vi "UI.vi"() -> ()   [LabVIEW 2016, in "潮位站数据传输.lvlib"]
panel:
  in  "记录报文":bool
  out "数据大小":i32
  out "数据上传中":bool
  out "当前时间":timestamp
  out "error out":errorcluster
  out "数据查表起始时间":T1
  in  "数据补传":bool caption="确定"
  out "读取报文显示":string
  out "发送报文显示":string
  out "通信状态":bool
  in  "配置信息":T2
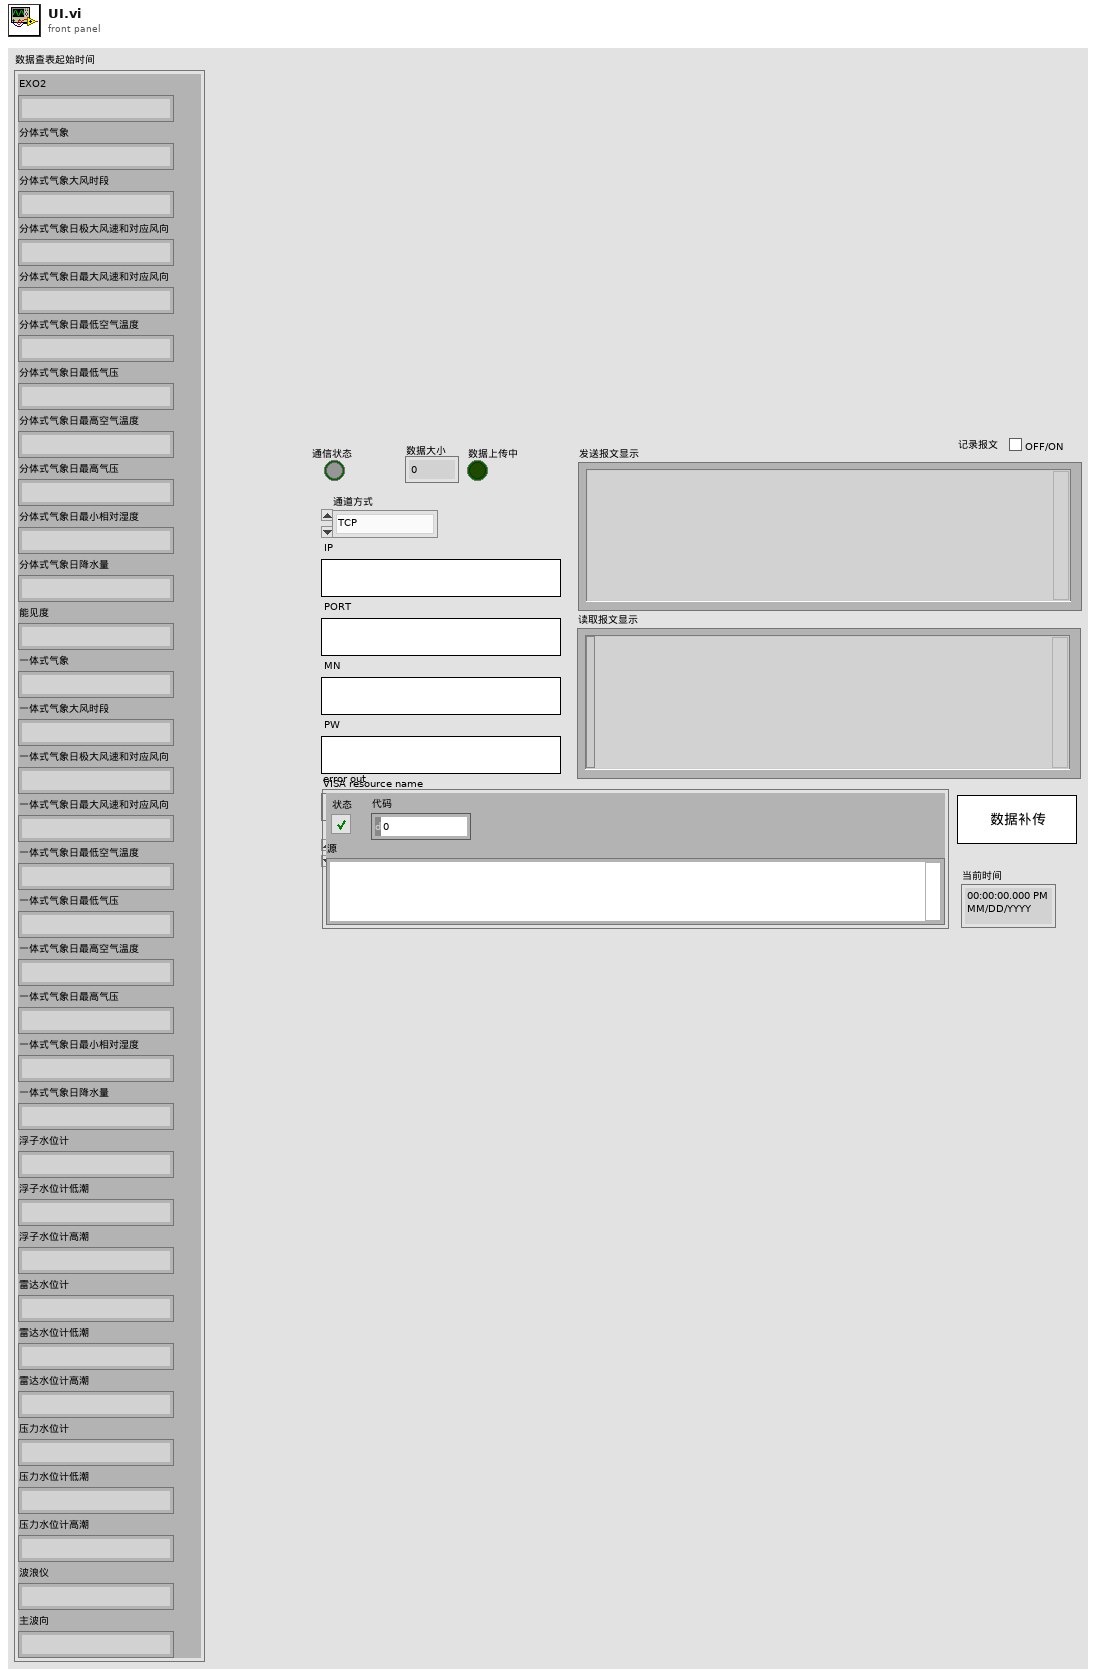
[diagram p1: front panel]
types:
  T1 = cluster{"EXO2":string, "分体式气象":string, "分体式气象大风时段":string, "分体式气象日极大风速和对应风向":string, "分体式气象日最大风速和对应风向":string, "分体式气象日最低空气温度":string, "分体式气象日最低气压":string, "分体式气象日最高空气温度":string, "分体式气象日最高气压":string, "分体式气象日最小相对湿度":string, "分体式气象日降水量":string, "能见度":string, "一体式气象":string, "一体式气象大风时段":string, "一体式气象日极大风速和对应风向":string, "一体式气象日最大风速和对应风向":string, "一体式气象日最低空气温度":string, "一体式气象日最低气压":string, "一体式气象日最高空气温度":string, "一体式气象日最高气压":string, "一体式气象日最小相对湿度":string, "一体式气象日降水量":string, "浮子水位计":string, "浮子水位计低潮":string, "浮子水位计高潮":string, "雷达水位计":string, "雷达水位计低潮":string, "雷达水位计高潮":string, "压力水位计":string, "压力水位计低潮":string, "压力水位计高潮":string, "波浪仪":string, "主波向":string}
  T2 = cluster{"通道方式":enum16{"TCP", "serial"}, "IP":string, "PORT":string, "MN":string, "PW":string, "VISA resource name":refnum<visa-resource-name>, "baud rate":u32}
  T3 = typedef "LVDateTimeRec.ctl" = cluster{"秒数的小数部分":dbl, "秒":i32, "分":i32, "时":i32, "日":i32, "月":i32, "年":i32, "天数（周）":i32, "天数（年）":i32, "DST":i32}
  T4 = cluster{"[0]":string, "[1]":string, "[2]":string, "[3]":string, "[4]":string, "[5]":string, "[6]":string, "[7]":string, "[8]":string, "[9]":string, "[10]":string, "[11]":string, "[12]":string, "[13]":string, "[14]":string, "[15]":string, "[16]":string, "[17]":string, "[18]":string, "[19]":string, "[20]":string, "[21]":string, "[22]":string, "[23]":string, "[24]":string, "[25]":string, "[26]":string, "[27]":string, "[28]":string, "[29]":string, "[30]":string, "[31]":string, "[32]":string}
  T5 = cluster{"枚举":enum16{"打开连接", "发送数据", "读取数据", "数据处理", "关闭连接"}, "data":string}
  T6 = cluster{"枚举":enum16{"TCP", "serial"}, "IP":string, "PORT":string, "MN":string, "PW":string, "VISA resource name":refnum<visa-resource-name>, "baud rate":u32}
  T7 = typedef "潮位站数据传输.lvlib/data_in.ctl" = cluster{"PW":string, "MN":string, "table输入":T8, "数据发送次数":i32, "枚举":enum16{"返回请求应答", "上传数据", "返回执行结果"}, "type":T9, "因子编码&数据类型":cluster{"因子编码":string, "数据类型":T10}[]}
  T8 = typedef "潮位站数据传输.lvlib/table.ctl" = string
  T9 = typedef "潮位站数据传输.lvlib/Type.ctl" = string
  T10 = typedef "潮位站数据传输.lvlib/data_type.ctl" = string
  T11 = cluster{"table":string, "columns":string[], "condition":string, "data_in":T7}
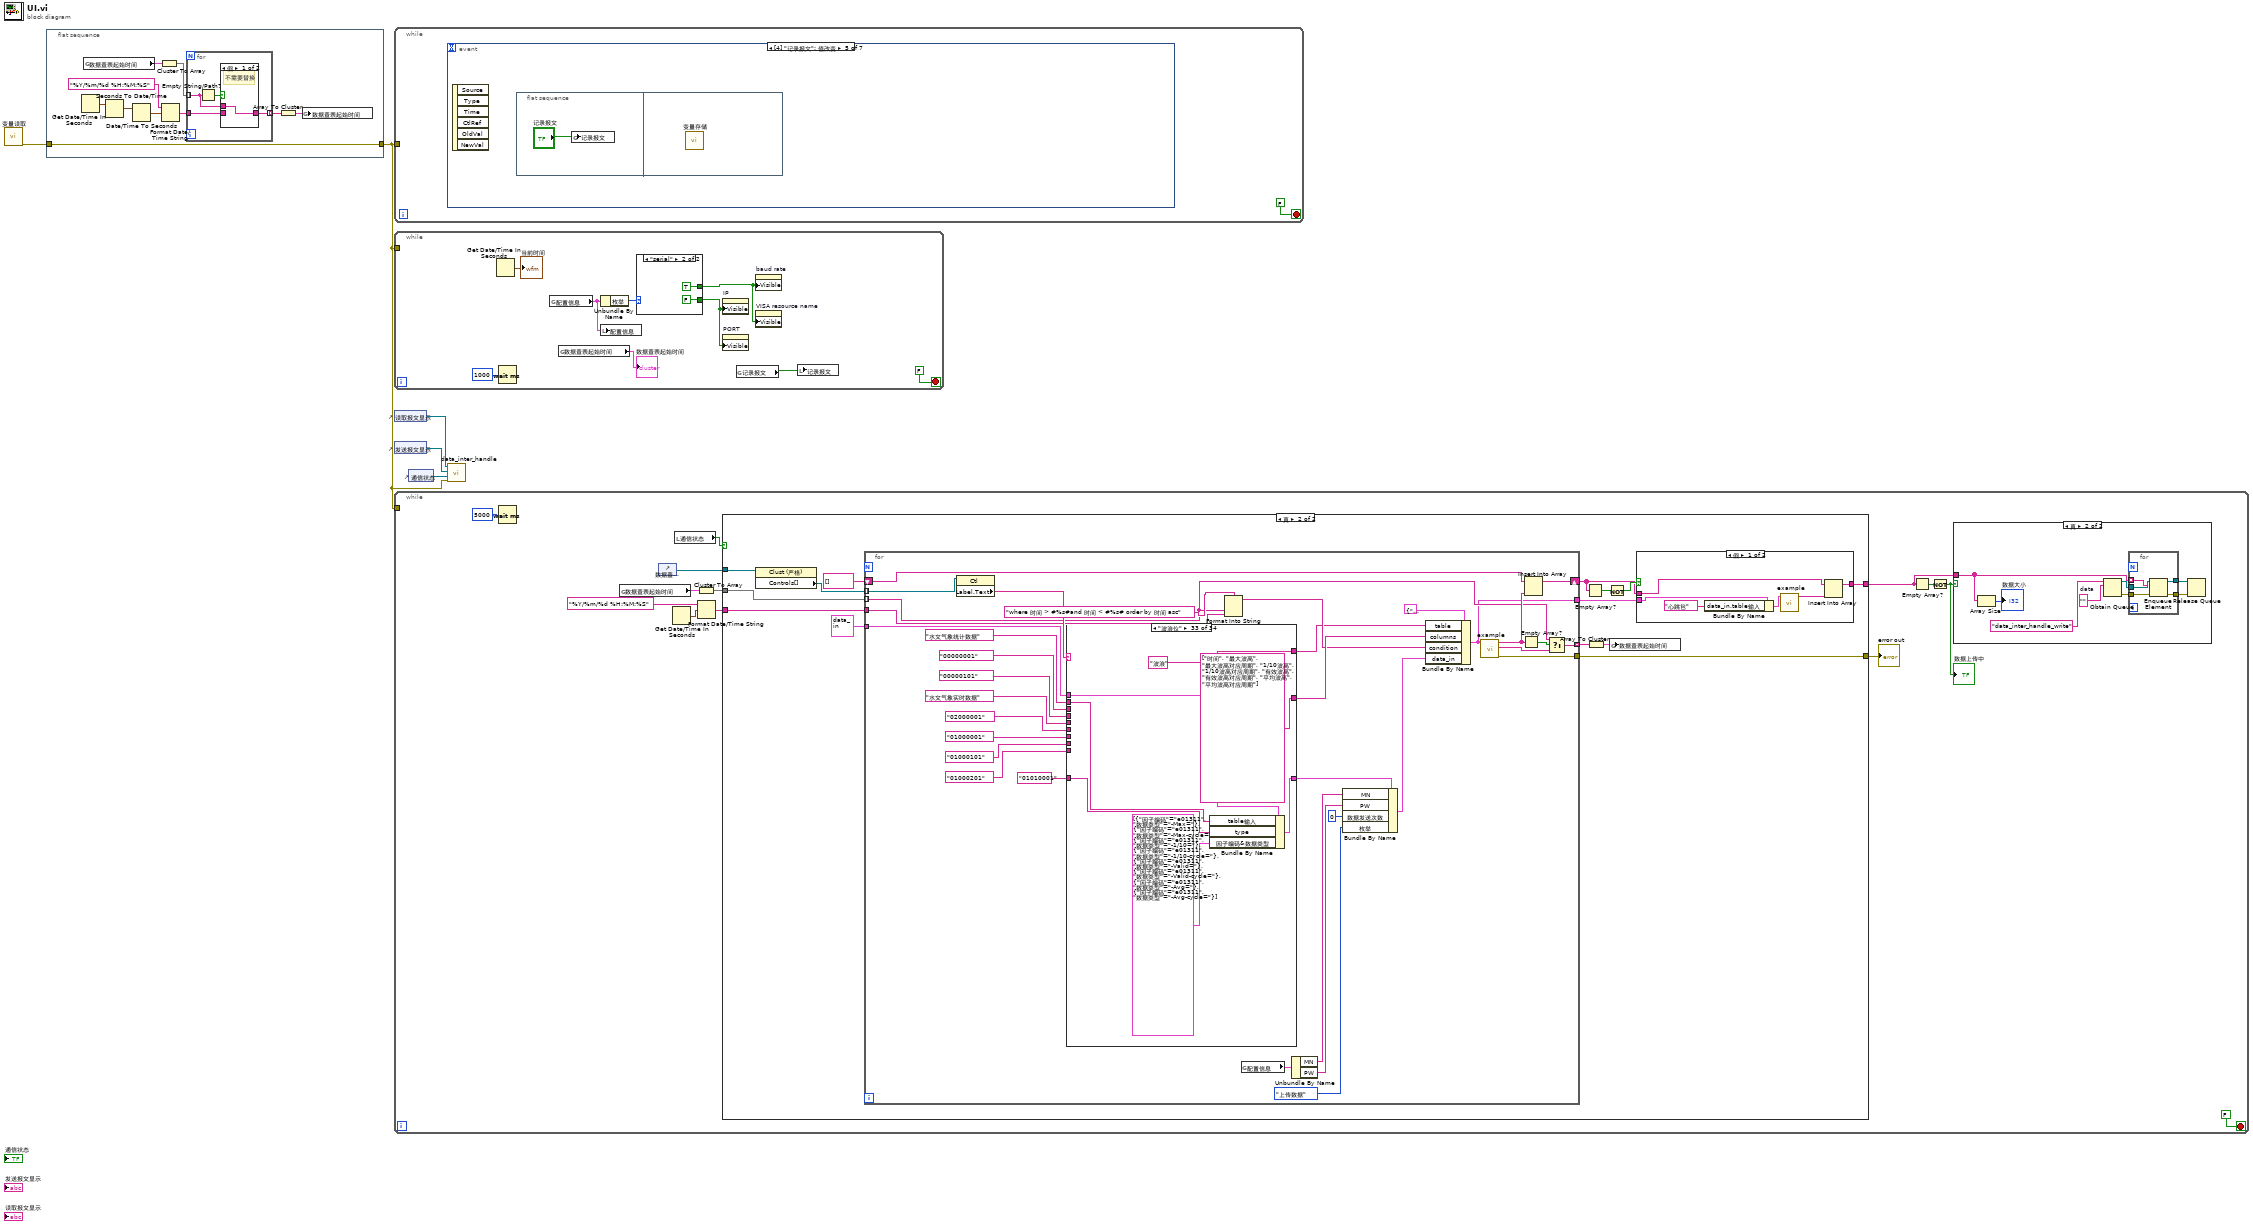
[diagram p0: block diagram]
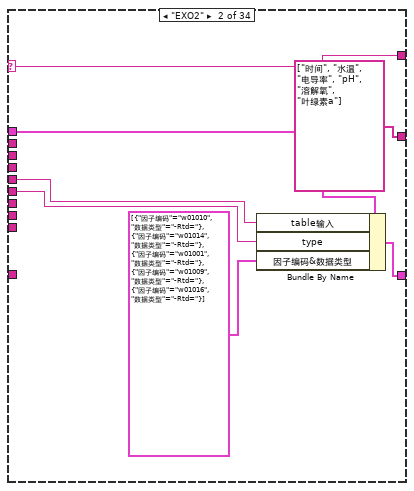
[diagram p6: hidden frame]
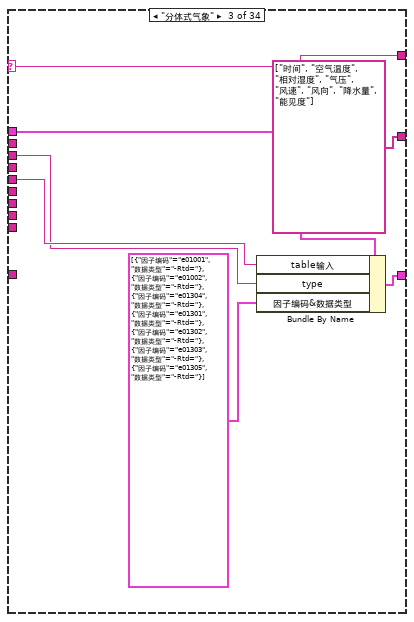
[diagram p7: hidden frame]
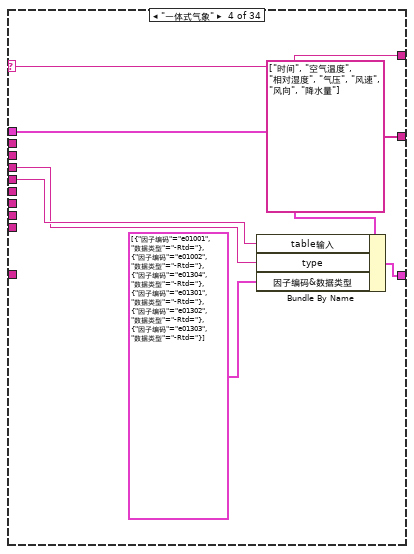
[diagram p8: hidden frame]
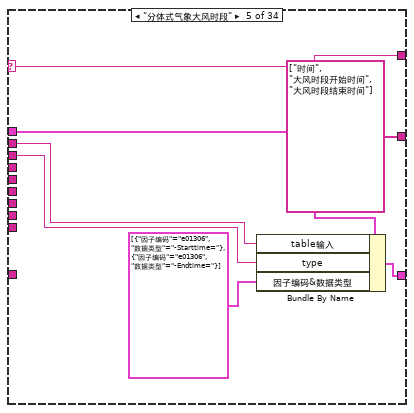
[diagram p9: hidden frame]
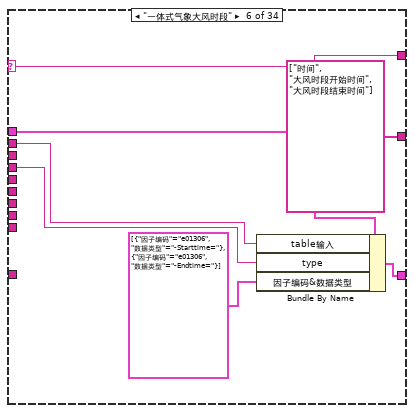
[diagram p10: hidden frame]
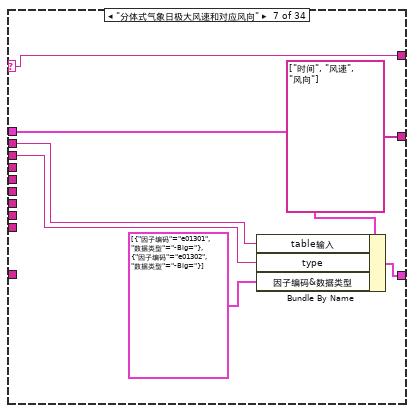
[diagram p11: hidden frame]
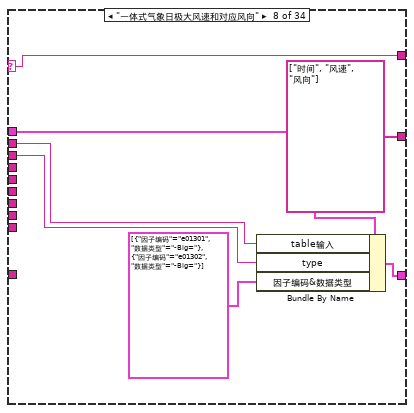
[diagram p12: hidden frame]
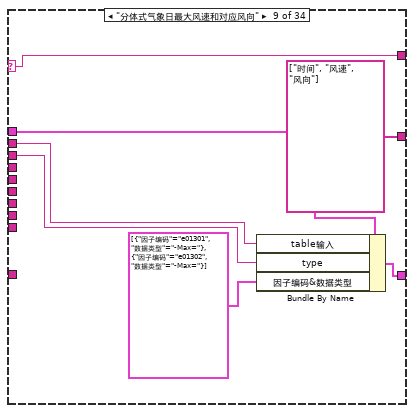
[diagram p13: hidden frame]
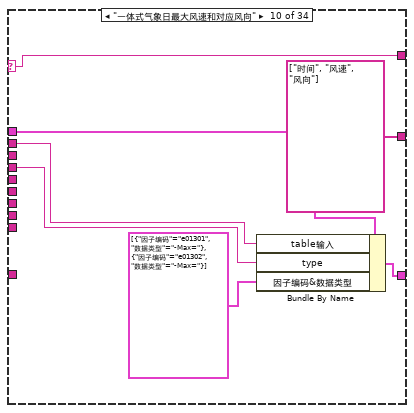
[diagram p14: hidden frame]
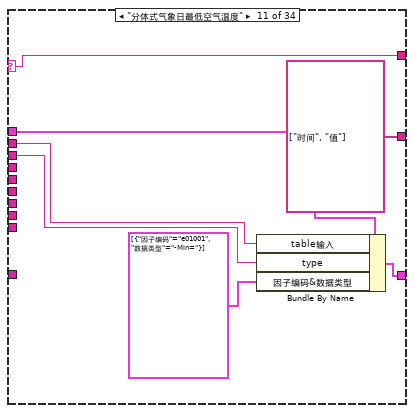
[diagram p15: hidden frame]
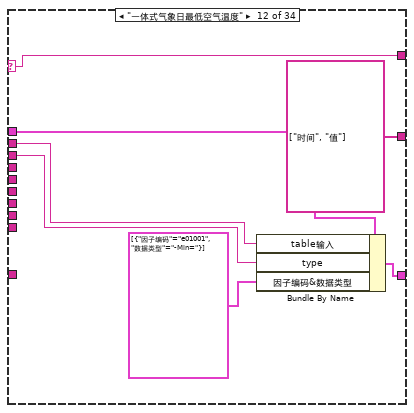
[diagram p16: hidden frame]
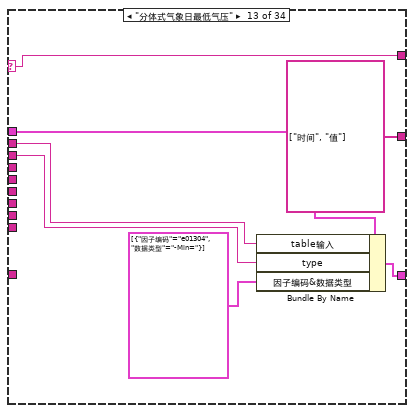
[diagram p17: hidden frame]
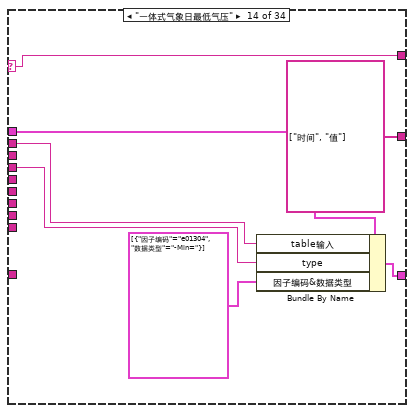
[diagram p18: hidden frame]
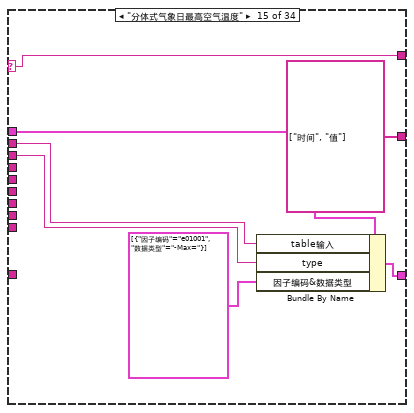
[diagram p19: hidden frame]
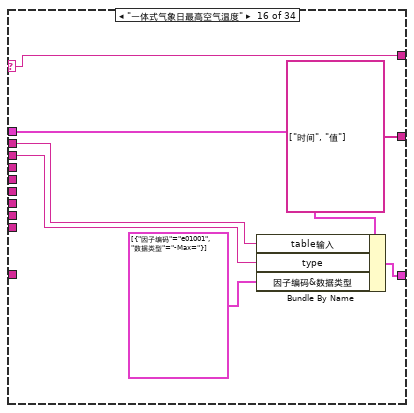
[diagram p20: hidden frame]
diagram:
  n1 = call "变量读取.vi"() -> ("错误输出"=w5:errorcluster)  [unwired: 11 in]
  n2 = flat-sequence {
    tunnel: w5 -> [w8]
    tunnel: [w8] -> w4
    frame #0 {
      n3 = Get Date/Time In Seconds() -> (seconds since 1Jan1904=w7:timestamp)
      n4 = global read "断电保存全局.vi" "数据查表起始时间"() -> (w13:T1)
      n5 = Seconds To Date/Time(time stamp (now)=w7) -> (date time rec=w6:T3)  [unwired: 1 in]
      n6 = Date/Time To Seconds(2:w6) -> (0:w11:timestamp)  [unwired: 1 in]
      n7 = Cluster To Array(cluster=w13) -> (array=w14:string[])
      n8 = Format Date/Time String(time format string (%c)="%Y/%m/%d %H:%M:%S" ("时间格式字符串(%c)"), seconds (now)=w11) -> (date/time string=w10:string)  [unwired: 1 in]
      n9 = for {
        tunnel: w14 -> [w16] mode=indexing
        tunnel: w10 -> [w18]
        tunnel: [w17] -> w15 mode=indexing
        n10 = Empty String/Path?(string/path=w16) -> (empty?=w19:bool)
        n11 = case shown="假" w19 {
          tunnel: w18 -> [_ w21]
          tunnel: [w20 w21] -> w17
          tunnel: w16 -> [w20 _]
          frame False {
            # "不需要替换"
          }
          frame True {
            # "空字符串，替换"
          }
        }
      }
      n12 = Array To Cluster(array=w15) -> (cluster=w9:T4)
      n13 = global write "断电保存全局.vi" "数据查表起始时间"(w9) -> ()
    }
  }
  n14 = while {
    tunnel: w4 -> [_]
    stop <- FALSE stop-if-true
    n15 = event shown="[4] \"记录报文\": 值改变" {
      selector: _ -> [_ _ _ _ _ _ _]
      dyn-events: _ -> [_ _ _ _ _ _ _]
      timeout: _ -> [_ _ _ _ _ _ _]
      event Timeout {
        n16 = event-data() -> ()  [unwired: 1 in, 3 out]
      }
      event "配置信息.IP", "配置信息.PORT": Mouse Down {
        n17 = event-data() -> ("CtlRef"=w31:refnum<vi>)  [unwired: 1 in, 7 out]
        n18 = property class="Str"(reference=w31) -> (reference out=w24:refnum<vi>, "Value"=w30:string)  [unwired: 1 in, 1 out]
        n19 = call "IP键盘.vi"("OldNumber"=w30) -> ("NewNumber"=w23:string)
        n20 = String Length(string=w23) -> (length=w29:i32)
        n21 = Less Or Equal?(x=w29, y=50) -> (x <= y?=w27:bool)
        n22 = case shown="假" w27 {
          tunnel: w24 -> [w32 w36]
          tunnel: w23 -> [_ w35]
          tunnel: [w32 w36] -> w26
          tunnel: ["127.0.0.1" w35] -> w25
          frame False {
            n23 = One Button Dialog(message="超过ipv4最大长度限制,请重新输入!" ("消息")) -> ()  [unwired: 1 in, 1 out]
          }
          frame True {
          }
        }
        n24 = property class="Str"(reference=w26, "Val(Sgnl)"=w25) -> ()  [unwired: 1 in, 2 out]
      }
      event "配置信息.baud rate": Mouse Down {
        n25 = event-data() -> ("CtlRef"=w40:refnum<vi>)  [unwired: 1 in, 7 out]
        n26 = property class="DigNum (严格)"(reference=w40) -> (reference out=w38:refnum<vi>, "Value"=w39:u32)  [unwired: 1 in, 1 out]
        n27 = call "数字键盘.vi"("OldNumber"=w39) -> ("NewNumber"=w37:sgl)
        n28 = property class="DigNum (严格)"(reference=w38, "Val(Sgnl)"=w37) -> ()  [unwired: 1 in, 2 out]
      }
      event "配置信息": Value Change {
        n29 = event-data() -> ()  [unwired: 1 in, 6 out]
        n30 = flat-sequence {
          frame #0 {
            n31 = global write "断电保存全局.vi" "配置信息"("配置信息") -> ()
          }
          frame #1 {
            w46 = T5 {"枚举"=enum."打开连接", "data"=""}
            n32 = call "变量存储.vi"() -> ()  [unwired: 12 in]
            n33 = Bundle By Name(cluster=w46, "枚举"=enum16{"打开连接", "发送数据", "读取数据", "数据处理", "关闭连接"}."关闭连接") -> (w45:T5)
            n34 = Obtain Queue(name (unnamed)="data_inter_handle" ("名称（未命名）"), element data type=w46) -> (queue out=w48:refnum<queue>, error out=w47:errorcluster)  [unwired: 3 in, 1 out]
            n35 = Enqueue Element(queue=w48, element=w45, error in (no error)=w47) -> (queue out=w42:refnum<queue>, error out=w43:errorcluster)  [unwired: 1 in, 1 out]
            n36 = Release Queue(queue=w42, error in (no error)=w43) -> ()  [unwired: 1 in, 3 out]
          }
        }
      }
      event "记录报文": Value Change {
        n37 = event-data() -> ()  [unwired: 1 in, 6 out]
        n38 = flat-sequence {
          frame #0 {
            n39 = global write "断电保存全局.vi" "记录报文"("记录报文") -> ()
          }
          frame #1 {
            n40 = call "变量存储.vi"() -> ()  [unwired: 12 in]
          }
        }
      }
      event "数据补传": Value Change {
        n41 = event-data() -> ()  [unwired: 1 in, 6 out]
        n42 = call "数据补传对话框.vi"() -> ("输出"=w52:bool, "时间OUT"=w51:timestamp)  [unwired: 10 in]
        n43 = case shown="真" w52 {
          tunnel: w51 -> [_ w57]
          frame False {
          }
          frame True {
            n44 = Format Date/Time String(time format string (%c)="%Y/%m/%d %H:%M:%S" ("时间格式字符串(%c)"), seconds (now)=w57) -> (date/time string=w54:string)  [unwired: 1 in]
            n45 = Initialize Array(w54, 33 ("维数大小")) -> (w53:string[])
            n46 = Array To Cluster(array=w53) -> (cluster=w55:T4)
            n47 = global write "断电保存全局.vi" "数据查表起始时间"(w55) -> ()
          }
        }
      }
      event Panel Close {
        n48 = event-data() -> ()  [unwired: 1 in, 4 out]
        n49 = Quit LabVIEW(quit? (T)=TRUE ("退出？(T)")) -> ()
      }
    }
  }
  n50 = while {
    tunnel: w4 -> [_]
    stop <- FALSE stop-if-true
    n51 = Get Date/Time In Seconds() -> (seconds since 1Jan1904=→"当前时间":timestamp)
    n52 = Wait (ms)(milliseconds to wait=u32 1000 ("等待时间（毫秒）")) -> ()  [unwired: 1 out]
    n53 = global read "断电保存全局.vi" "配置信息"() -> (w64:T6)
    n54 = global read "断电保存全局.vi" "数据查表起始时间"() -> (→"数据查表起始时间":T1)
    n55 = local write "配置信息"(w64) -> ()
    n56 = Unbundle By Name(w64) -> ("枚举"=w63:enum16{"TCP", "serial"})
    n57 = case shown="\"serial\"" w63 {
      tunnel: [TRUE FALSE] -> w62
      tunnel: [FALSE TRUE] -> w61
      frame "TCP", Default {
      }
      frame "serial" {
      }
    }
    n58 = property on="IP" class="Str"("Visible"=w62) -> ()  [unwired: 2 in, 2 out]
    n59 = property on="PORT" class="Str"("Visible"=w62) -> ()  [unwired: 2 in, 2 out]
    n60 = global read "断电保存全局.vi" "记录报文"() -> (w60:bool)
    n61 = property on="baud rate" class="DigNum (严格)"("Visible"=w61) -> ()  [unwired: 2 in, 2 out]
    n62 = property on="VISA resource name" class="VISAName"("Visible"=w61) -> ()  [unwired: 2 in, 2 out]
    n63 = local write "记录报文"(w60) -> ()
  }
  n64 = control-ref of="读取报文显示"() -> (w2:refnum<vi>)
  n65 = control-ref of="发送报文显示"() -> (w3:refnum<vi>)
  n66 = while {
    tunnel: w4 -> [_]
    stop <- FALSE stop-if-true
    n67 = Wait (ms)(milliseconds to wait=u32 5000 ("等待时间（毫秒）")) -> ()  [unwired: 1 out]
    n68 = global read "断电保存全局.vi" "数据查表起始时间"() -> (w83:T1)
    n69 = control-ref of="数据查表起始时间"() -> (w77:refnum<vi>)
    n70 = Get Date/Time In Seconds() -> (seconds since 1Jan1904=w79:timestamp)
    n71 = local read "通信状态"() -> (w74:bool)
    n72 = Cluster To Array(cluster=w83) -> (array=w82:string[])
    n73 = Format Date/Time String(time format string (%c)="%Y/%m/%d %H:%M:%S" ("时间格式字符串(%c)"), seconds (now)=w79) -> (date/time string=w80:string)  [unwired: 1 in]
    n74 = case shown="真" w74 {
      tunnel: w82 -> [_ w99]
      tunnel: w80 -> [_ w98]
      tunnel: [_ w87] -> w73
      tunnel: w77 -> [_ w97]
      tunnel: [_ w95] -> w76
      frame False {
      }
      frame True {
        n75 = property class="Clust (严格)"(reference=w97) -> ("Controls[]"=w96:refnum<vi>[])  [unwired: 1 in, 2 out]
        n76 = for {
          tunnel: w99 -> [w124] mode=indexing
          tunnel: w96 -> [w140] mode=indexing
          tunnel: w98 -> [w130]
          shift-right: [w127] -> w88
          shift-left: string[] [] ("message") -> [w128]
          tunnel: [w122] -> w92 mode=indexing
          tunnel: [w121] -> w95
          tunnel: T7 {"PW"="123456", "MN"="TEST001", "table输入"="心跳包", "数据发送次数"=0, "枚举"=enum."上传数据", "type"="00000001", "因子编码&数据类型"=[{"因子编码"="e01306", "数据类型"="-Starttime="}, {"因子编码"="e01307", "数据类型"="-Endtime="}]} ("data_in") -> [w119]
          tunnel: [w110] -> w86
          n77 = property class="Ctl"(reference=w140) -> ("Label.Text"=w139:string)  [unwired: 1 in, 2 out]
          n78 = case shown="\"波浪仪\"" w139 {
            selector: w139 -> [w141 w142 w149 w156 w163 w170 w177 w184 w191 w198 w205 w212 w219 w226 w233 w240 w247 w254 w261 w268 w275 w282 w289 w296 w303 w310 w317 w324 w331 w338 w345 w352 _ _]
            tunnel: [_ string[] ["时间", "水温", "电导率", "pH", "溶解氧", "叶绿素a"] ("columns") string[] ["时间", "空气温度", "相对湿度", "气压", "风速", "风向", "降水量", "能见度"] ("columns") string[] ["时间", "空气温度", "相对湿度", "气压", "风速", "风向", "降水量"] ("columns") string[] ["时间", "大风时段开始时间", "大风时段结束时间"] ("columns") string[] ["时间", "大风时段开始时间", "大风时段结束时间"] ("columns") string[] ["时间", "风速", "风向"] ("columns") string[] ["时间", "风速", "风向"] ("columns") string[] ["时间", "风速", "风向"] ("columns") string[] ["时间", "风速", "风向"] ("columns") string[] ["时间", "值"] ("columns") string[] ["时间", "值"] ("columns") string[] ["时间", "值"] ("columns") string[] ["时间", "值"] ("columns") string[] ["时间", "值"] ("columns") string[] ["时间", "值"] ("columns") string[] ["时间", "值"] ("columns") string[] ["时间", "值"] ("columns") string[] ["时间", "值"] ("columns") string[] ["时间", "值"] ("columns") string[] ["时间", "值"] ("columns") string[] ["时间", "值"] ("columns") string[] ["时间", "60秒能见度"] ("columns") string[] ["时间", "潮高"] ("columns") string[] ["时间", "潮高"] ("columns") string[] ["时间", "潮高"] ("columns") string[] ["时间", "潮高"] ("columns") string[] ["时间", "潮高"] ("columns") string[] ["时间", "潮高"] ("columns") string[] ["时间", "潮高"] ("columns") string[] ["时间", "潮高"] ("columns") string[] ["时间", "潮高"] ("columns") string[] ["时间", "最大波高", "最大波高对应周期", "1/10波高", "1/10波高对应周期", "有效波高", "有效波高对应周期", "平均波高", "平均波高对应周期"] ("columns") string[] ["时间", "主波向"] ("columns")] -> w138
            tunnel: w119 -> [_ w147 w154 w161 w168 w175 w182 w189 w196 w203 w210 w217 w224 w231 w238 w245 w252 w259 w266 w273 w280 w287 w294 w301 w308 w315 w322 w329 w336 w343 w350 w357 w364 w372]
            tunnel: [_ w146 w153 w160 w167 w174 w181 w188 w195 w202 w209 w216 w223 w230 w237 w244 w251 w258 w265 w272 w279 w286 w293 w300 w307 w314 w321 w328 w335 w342 w349 w356 w363 w371] -> w108
            tunnel: T9 "00000001" ("type") -> [_ _ w150 _ w165 _ w179 w185 w193 _ w207 w214 w221 _ w235 w242 w249 _ w263 _ w276 _ w290 _ _ _ _ _ _ _ _ _ _ _]
            tunnel: T9 "00000101" ("type") -> [_ _ _ w157 _ w171 _ _ _ w200 _ _ _ w228 _ _ _ w256 _ w270 _ w284 _ _ _ _ _ _ _ _ _ _ _ _]
            tunnel: T9 "01000001" ("type") -> [_ _ _ _ _ _ _ _ _ _ _ _ _ _ _ _ _ _ _ _ _ _ _ w298 _ _ w318 _ _ w340 _ _ _ _]
            tunnel: T9 "01000101" ("type") -> [_ _ _ _ _ _ _ _ _ _ _ _ _ _ _ _ _ _ _ _ _ _ _ _ w305 _ _ w326 _ _ w346 _ _ _]
            tunnel: T9 "01000201" ("type") -> [_ _ _ _ _ _ _ _ _ _ _ _ _ _ _ _ _ _ _ _ _ _ _ _ _ w312 _ _ w332 _ _ w354 _ _]
            tunnel: T9 "02000001" ("type") -> [_ w143 _ _ _ _ _ _ _ _ _ _ _ _ _ _ _ _ _ _ _ _ _ _ _ _ _ _ _ _ _ _ _ _]
            tunnel: T8 "水文气象实时数据" ("table输入") -> [_ w144 w151 w158 _ _ _ _ _ _ _ _ _ _ _ _ _ _ _ _ _ _ w291 w297 w304 w311 _ _ _ _ _ _ _ w367]
            tunnel: T8 "水文气象统计数据" ("table输入") -> [_ _ _ _ w164 w172 w178 w186 w192 w199 w206 w213 w220 w227 w234 w241 w248 w255 w262 w269 w277 w283 _ _ _ _ w319 w325 w333 w339 w347 w353 w361 _]
            tunnel: T9 "01010001" ("type") -> [_ _ _ _ _ _ _ _ _ _ _ _ _ _ _ _ _ _ _ _ _ _ _ _ _ _ _ _ _ _ _ _ w360 w369]
            tunnel: [w141 w142 w149 w156 w163 w170 w177 w184 w191 w198 w205 w212 w219 w226 w233 w240 w247 w254 w261 w268 w275 w282 w289 w296 w303 w310 w317 w324 w331 w338 w345 w352 "波浪" "波浪"] -> w107
            frame "假", Default {
            }
            frame "EXO2" {
              n79 = Bundle By Name(cluster=w147, "table输入"=w144, "type"=w143, "因子编码&数据类型"=cluster{"因子编码":string, "数据类型":string}[] [{"因子编码"="w01010", "数据类型"="-Rtd="}, {"因子编码"="w01014", "数据类型"="-Rtd="}, {"因子编码"="w01001", "数据类型"="-Rtd="}, {"因子编码"="w01009", "数据类型"="-Rtd="}, {"因子编码"="w01016", "数据类型"="-Rtd="}]) -> (w146:T7)
            }
            frame "分体式气象" {
              n80 = Bundle By Name(cluster=w154, "table输入"=w151, "type"=w150, "因子编码&数据类型"=cluster{"因子编码":string, "数据类型":string}[] [{"因子编码"="e01001", "数据类型"="-Rtd="}, {"因子编码"="e01002", "数据类型"="-Rtd="}, {"因子编码"="e01304", "数据类型"="-Rtd="}, {"因子编码"="e01301", "数据类型"="-Rtd="}, {"因子编码"="e01302", "数据类型"="-Rtd="}, {"因子编码"="e01303", "数据类型"="-Rtd="}, {"因子编码"="e01305", "数据类型"="-Rtd="}]) -> (w153:T7)
            }
            frame "一体式气象" {
              n81 = Bundle By Name(cluster=w161, "table输入"=w158, "type"=w157, "因子编码&数据类型"=cluster{"因子编码":string, "数据类型":string}[] [{"因子编码"="e01001", "数据类型"="-Rtd="}, {"因子编码"="e01002", "数据类型"="-Rtd="}, {"因子编码"="e01304", "数据类型"="-Rtd="}, {"因子编码"="e01301", "数据类型"="-Rtd="}, {"因子编码"="e01302", "数据类型"="-Rtd="}, {"因子编码"="e01303", "数据类型"="-Rtd="}]) -> (w160:T7)
            }
            frame "分体式气象大风时段" {
              n82 = Bundle By Name(cluster=w168, "table输入"=w164, "type"=w165, "因子编码&数据类型"=cluster{"因子编码":string, "数据类型":string}[] [{"因子编码"="e01306", "数据类型"="-Starttime="}, {"因子编码"="e01306", "数据类型"="-Endtime="}]) -> (w167:T7)
            }
            frame "一体式气象大风时段" {
              n83 = Bundle By Name(cluster=w175, "table输入"=w172, "type"=w171, "因子编码&数据类型"=cluster{"因子编码":string, "数据类型":string}[] [{"因子编码"="e01306", "数据类型"="-Starttime="}, {"因子编码"="e01306", "数据类型"="-Endtime="}]) -> (w174:T7)
            }
            frame "分体式气象日极大风速和对应风向" {
              n84 = Bundle By Name(cluster=w182, "table输入"=w178, "type"=w179, "因子编码&数据类型"=cluster{"因子编码":string, "数据类型":string}[] [{"因子编码"="e01301", "数据类型"="-Big="}, {"因子编码"="e01302", "数据类型"="-Big="}]) -> (w181:T7)
            }
            frame "一体式气象日极大风速和对应风向" {
              n85 = Bundle By Name(cluster=w189, "table输入"=w186, "type"=w185, "因子编码&数据类型"=cluster{"因子编码":string, "数据类型":string}[] [{"因子编码"="e01301", "数据类型"="-Big="}, {"因子编码"="e01302", "数据类型"="-Big="}]) -> (w188:T7)
            }
            frame "分体式气象日最大风速和对应风向" {
              n86 = Bundle By Name(cluster=w196, "table输入"=w192, "type"=w193, "因子编码&数据类型"=cluster{"因子编码":string, "数据类型":string}[] [{"因子编码"="e01301", "数据类型"="-Max="}, {"因子编码"="e01302", "数据类型"="-Max="}]) -> (w195:T7)
            }
            frame "一体式气象日最大风速和对应风向" {
              n87 = Bundle By Name(cluster=w203, "table输入"=w199, "type"=w200, "因子编码&数据类型"=cluster{"因子编码":string, "数据类型":string}[] [{"因子编码"="e01301", "数据类型"="-Max="}, {"因子编码"="e01302", "数据类型"="-Max="}]) -> (w202:T7)
            }
            frame "分体式气象日最低空气温度" {
              n88 = Bundle By Name(cluster=w210, "table输入"=w206, "type"=w207, "因子编码&数据类型"=cluster{"因子编码":string, "数据类型":string}[] [{"因子编码"="e01001", "数据类型"="-Min="}]) -> (w209:T7)
            }
            frame "一体式气象日最低空气温度" {
              n89 = Bundle By Name(cluster=w217, "table输入"=w213, "type"=w214, "因子编码&数据类型"=cluster{"因子编码":string, "数据类型":string}[] [{"因子编码"="e01001", "数据类型"="-Min="}]) -> (w216:T7)
            }
            frame "分体式气象日最低气压" {
              n90 = Bundle By Name(cluster=w224, "table输入"=w220, "type"=w221, "因子编码&数据类型"=cluster{"因子编码":string, "数据类型":string}[] [{"因子编码"="e01304", "数据类型"="-Min="}]) -> (w223:T7)
            }
            frame "一体式气象日最低气压" {
              n91 = Bundle By Name(cluster=w231, "table输入"=w227, "type"=w228, "因子编码&数据类型"=cluster{"因子编码":string, "数据类型":string}[] [{"因子编码"="e01304", "数据类型"="-Min="}]) -> (w230:T7)
            }
            frame "分体式气象日最高空气温度" {
              n92 = Bundle By Name(cluster=w238, "table输入"=w234, "type"=w235, "因子编码&数据类型"=cluster{"因子编码":string, "数据类型":string}[] [{"因子编码"="e01001", "数据类型"="-Max="}]) -> (w237:T7)
            }
            frame "一体式气象日最高空气温度" {
              n93 = Bundle By Name(cluster=w245, "table输入"=w241, "type"=w242, "因子编码&数据类型"=cluster{"因子编码":string, "数据类型":string}[] [{"因子编码"="e01001", "数据类型"="-Max="}]) -> (w244:T7)
            }
            frame "分体式气象日最高气压" {
              n94 = Bundle By Name(cluster=w252, "table输入"=w248, "type"=w249, "因子编码&数据类型"=cluster{"因子编码":string, "数据类型":string}[] [{"因子编码"="e01304", "数据类型"="-Max="}]) -> (w251:T7)
            }
            frame "一体式气象日最高气压" {
              n95 = Bundle By Name(cluster=w259, "table输入"=w255, "type"=w256, "因子编码&数据类型"=cluster{"因子编码":string, "数据类型":string}[] [{"因子编码"="e01304", "数据类型"="-Max="}]) -> (w258:T7)
            }
            frame "分体式气象日最小相对湿度" {
              n96 = Bundle By Name(cluster=w266, "table输入"=w262, "type"=w263, "因子编码&数据类型"=cluster{"因子编码":string, "数据类型":string}[] [{"因子编码"="e01002", "数据类型"="-Min="}]) -> (w265:T7)
            }
            frame "一体式气象日最小相对湿度" {
              n97 = Bundle By Name(cluster=w273, "table输入"=w269, "type"=w270, "因子编码&数据类型"=cluster{"因子编码":string, "数据类型":string}[] [{"因子编码"="e01002", "数据类型"="-Min="}]) -> (w272:T7)
            }
            frame "分体式气象日降水量" {
              n98 = Bundle By Name(cluster=w280, "table输入"=w277, "type"=w276, "因子编码&数据类型"=cluster{"因子编码":string, "数据类型":string}[] [{"因子编码"="e01303", "数据类型"="-Day="}]) -> (w279:T7)
            }
            frame "一体式气象日降水量" {
              n99 = Bundle By Name(cluster=w287, "table输入"=w283, "type"=w284, "因子编码&数据类型"=cluster{"因子编码":string, "数据类型":string}[] [{"因子编码"="e01303", "数据类型"="-Day="}]) -> (w286:T7)
            }
            frame "能见度" {
              n100 = Bundle By Name(cluster=w294, "table输入"=w291, "type"=w290, "因子编码&数据类型"=cluster{"因子编码":string, "数据类型":string}[] [{"因子编码"="e01305", "数据类型"="-Rtd="}]) -> (w293:T7)
            }
            frame "浮子水位计" {
              n101 = Bundle By Name(cluster=w301, "table输入"=w297, "type"=w298, "因子编码&数据类型"=cluster{"因子编码":string, "数据类型":string}[] [{"因子编码"="e01308", "数据类型"="-Rtd="}]) -> (w300:T7)
            }
            frame "雷达水位计" {
              n102 = Bundle By Name(cluster=w308, "table输入"=w304, "type"=w305, "因子编码&数据类型"=cluster{"因子编码":string, "数据类型":string}[] [{"因子编码"="e01308", "数据类型"="-Rtd="}]) -> (w307:T7)
            }
            frame "压力水位计" {
              n103 = Bundle By Name(cluster=w315, "table输入"=w311, "type"=w312, "因子编码&数据类型"=cluster{"因子编码":string, "数据类型":string}[] [{"因子编码"="e01308", "数据类型"="-Rtd="}]) -> (w314:T7)
            }
            frame "浮子水位计低潮" {
              n104 = Bundle By Name(cluster=w322, "table输入"=w319, "type"=w318, "因子编码&数据类型"=cluster{"因子编码":string, "数据类型":string}[] [{"因子编码"="e01310", "数据类型"="-Trough="}]) -> (w321:T7)
            }
            frame "雷达水位计低潮" {
              n105 = Bundle By Name(cluster=w329, "table输入"=w325, "type"=w326, "因子编码&数据类型"=cluster{"因子编码":string, "数据类型":string}[] [{"因子编码"="e01310", "数据类型"="-Trough="}]) -> (w328:T7)
            }
            frame "压力水位计低潮" {
              n106 = Bundle By Name(cluster=w336, "table输入"=w333, "type"=w332, "因子编码&数据类型"=cluster{"因子编码":string, "数据类型":string}[] [{"因子编码"="e01310", "数据类型"="-Trough="}]) -> (w335:T7)
            }
            frame "浮子水位计高潮" {
              n107 = Bundle By Name(cluster=w343, "table输入"=w339, "type"=w340, "因子编码&数据类型"=cluster{"因子编码":string, "数据类型":string}[] [{"因子编码"="e01309", "数据类型"="-Peak="}]) -> (w342:T7)
            }
            frame "雷达水位计高潮" {
              n108 = Bundle By Name(cluster=w350, "table输入"=w347, "type"=w346, "因子编码&数据类型"=cluster{"因子编码":string, "数据类型":string}[] [{"因子编码"="e01309", "数据类型"="-Peak="}]) -> (w349:T7)
            }
            frame "压力水位计高潮" {
              n109 = Bundle By Name(cluster=w357, "table输入"=w353, "type"=w354, "因子编码&数据类型"=cluster{"因子编码":string, "数据类型":string}[] [{"因子编码"="e01309", "数据类型"="-Peak="}]) -> (w356:T7)
            }
            frame "波浪仪" {
              n110 = Bundle By Name(cluster=w364, "table输入"=w361, "type"=w360, "因子编码&数据类型"=cluster{"因子编码":string, "数据类型":T10}[] [{"因子编码"="e01311", "数据类型"="-Max="}, {"因子编码"="e01311", "数据类型"="-Max-cycle="}, {"因子编码"="e01311", "数据类型"="-1/10="}, {"因子编码"="e01311", "数据类型"="-1/10-cycle="}, {"因子编码"="e01311", "数据类型"="-Valid="}, {"因子编码"="e01311", "数据类型"="-Valid-cycle="}, {"因子编码"="e01311", "数据类型"="-Avg="}, {"因子编码"="e01311", "数据类型"="-Avg-cycle="}]) -> (w363:T7)
            }
            frame "主波向" {
              n111 = Bundle By Name(cluster=w372, "table输入"=w367, "type"=w369, "因子编码&数据类型"=cluster{"因子编码":string, "数据类型":T10}[] [{"因子编码"="e01312", "数据类型"="-Rtd="}]) -> (w371:T7)
            }
          }
          n112 = Format Into String(format string="where 时间 > #%s#and 时间 < #%s# order by 时间 asc" ("初始字符串"), w124, w130) -> (resulting string=w129:string)  [unwired: 2 in, 1 out]
          n113 = global read "断电保存全局.vi" "配置信息"() -> (w137:T6)
          n114 = Unbundle By Name(w137) -> ("MN"=w136:string, "PW"=w135:string)
          n115 = Bundle By Name(cluster=w108, "MN"=w136, "PW"=w135, "数据发送次数"=0, "枚举"=enum16{"返回请求应答", "上传数据", "返回执行结果"}."上传数据") -> (w132:T7)
          n116 = Bundle By Name(cluster=T11 {"table"="分体式气象大风时段", "columns"=["时间", "大风时段开始时间", "大风时段结束时间"], "condition"="", "data_in"={"PW"="123456", "MN"="TEST001", "table输入"="心跳包", "数据发送次数"=0, "枚举"=enum."上传数据", "type"="00000001", "因子编码&数据类型"=[{"因子编码"="e01306", "数据类型"="-Starttime="}, {"因子编码"="e01307", "数据类型"="-Endtime="}]}} ("data_in"), "table"=w107, "columns"=w138, "condition"=w129, "data_in"=w132) -> (w110:T11)
          n117 = call "example.vi"("data_in"=w110) -> ("error out"=w121:errorcluster, "最新时间"=w123:string, "message"=w126:string[])  [unwired: 8 in]
          n118 = Empty Array?(array=w126) -> (empty?=w125:bool)
          n119 = Insert Into Array(array=w128, new element=w126) -> (w127:string[])  [unwired: 1 in]
          n120 = Select(t=w124, s=w125, f=w123) -> (s? t:f=w122:string)
        }
        n121 = Empty Array?(array=w88) -> (empty?=w90:bool)
        n122 = Array To Cluster(array=w92) -> (cluster=w93:T4)
        n123 = Not(x=w90) -> (.not. x?=w89:bool)
        n124 = global write "断电保存全局.vi" "数据查表起始时间"(w93) -> ()
        n125 = case shown="假" w89 {
          tunnel: w88 -> [w102 w106]
          tunnel: [w100 w106] -> w87
          tunnel: w86 -> [w105 _]
          frame False {
            n126 = Bundle By Name(cluster=w105, "data_in.table输入"=T8 "心跳包") -> (w103:T11)
            n127 = call "example.vi"("data_in"=w103) -> ("message"=w101:string[])  [unwired: 8 in, 2 out]
            n128 = Insert Into Array(array=w102, new element=w101) -> (w100:string[])  [unwired: 1 in]
          }
          frame True {
          }
        }
      }
    }
    "error out" <- w76
    n129 = Empty Array?(array=w73) -> (empty?=w78:bool)
    n130 = Not(x=w78) -> (.not. x?=w75:bool)
    "数据上传中" <- w75
    n131 = case shown="真" w75 {
      tunnel: w73 -> [_ w373]
      frame False {
      }
      frame True {
        w375 = ""  # data
        n132 = Array Size(array=w373) -> (size(s)=→"数据大小":i32)
        n133 = Obtain Queue(name (unnamed)="data_inter_handle_write" ("名称（未命名）"), element data type=w375) -> (queue out=w380:refnum<queue>, error out=w379:errorcluster)  [unwired: 3 in, 1 out]
        n134 = for {
          tunnel: w380 -> [w385]
          tunnel: w379 -> [w384]
          tunnel: [w383] -> w378
          tunnel: [w382] -> w377
          tunnel: w373 -> [w381] mode=indexing
          n135 = Enqueue Element(queue=w385, element=w381, error in (no error)=w384) -> (queue out=w383:refnum<queue>, error out=w382:errorcluster)  [unwired: 1 in, 1 out]
        }
        n136 = Release Queue(queue=w378, error in (no error)=w377) -> ()  [unwired: 1 in, 3 out]
      }
    }
  }
  n137 = control-ref of="通信状态"() -> (w1:refnum<vi>)
  n138 = call "data_inter_handle.vi"("error in (no error)"=w4, "通信状态"=w1, "发送报文显示"=w3, "读取报文显示"=w2) -> ()  [unwired: 7 in, 1 out]
